vi "ProcessControl-WaitOnStop.vi"(2 "PROCESS":string, 9 "error out":errorcluster caption="error in (no error)") -> (6 "error in":errorcluster caption="error out")   [LabVIEW 2009]
uses:
  ProcessControl.ctl
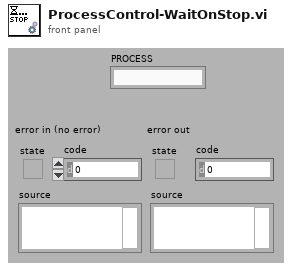
[diagram p1: front panel]
types:
  T1 = typedef "ProcessControl.ctl" = enum16{"STOP"}
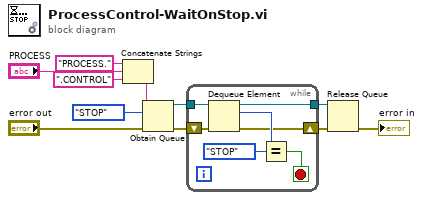
[diagram p0: block diagram]
diagram:
  n1 = Concatenate Strings("PROCESS." ("chaîne"), "PROCESS", ".CONTROL" ("chaîne")) -> (w3:string)
  n2 = Obtain Queue(name (unnamed)=w3, element data type=ProcessControl."STOP" ("ProcessControl"), error in (no error)="error out") -> (queue out=w5:refnum<queue>, error out=w6:errorcluster)  [unwired: 2 in, 1 out]
  n3 = while {
    tunnel: w5 -> [w18]
    tunnel: [w14] -> w8
    shift-right: [w13] -> w7
    shift-left: w6 -> [w17]
    stop <- w12 stop-if-true
    n4 = Dequeue Element(queue=w18, error in (no error)=w17) -> (queue out=w14:refnum<queue>, element=w15:T1, error out=w13:errorcluster)  [unwired: 2 out]
    n5 = Equal?(x=w15, y=ProcessControl."STOP" ("ProcessControl")) -> (x = y?=w12:bool)
  }
  n6 = Release Queue(queue=w8, error in (no error)=w7) -> (error out=→"error in":errorcluster)  [unwired: 3 out]
